vi "SR1.vi"(1 "Spoken text box":refnum<vi>, 2 "new reference":refnum<k24>) -> (0 "事件回调":refnum<k27>)   [LabVIEW 2009]
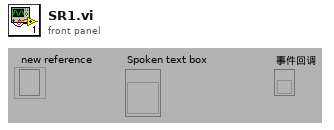
[diagram p1: front panel]
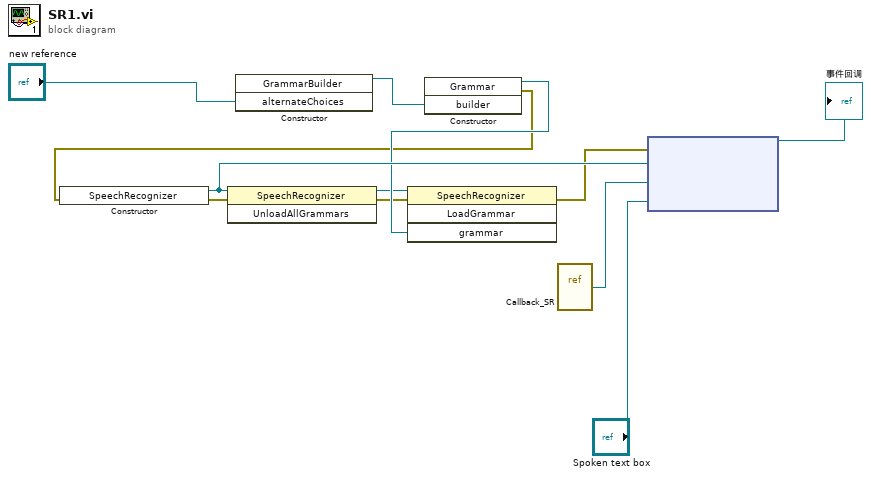
[diagram p0: block diagram]
diagram:
  n1 = constructor class="GrammarBuilder"("alternateChoices"="new reference") -> (reference out=w2:refnum<k24>)  [unwired: 3 in, 3 out]
  n2 = constructor class="Grammar"("builder"=w2) -> (reference out=w7:refnum<k24>, error out=w4:errorcluster)  [unwired: 3 in, 2 out]
  n3 = constructor class="SpeechRecognizer"(error in=w4) -> (reference out=w12:refnum<k24>, error out=w3:errorcluster)  [unwired: 2 in, 1 out]
  n4 = invoke class="SpeechRecognizer" method="UnloadAllGrammars"(reference=w12, error in=w3) -> (reference out=w5:refnum<k24>, error out=w6:errorcluster)  [unwired: 1 in, 1 out]
  n5 = invoke class="SpeechRecognizer" method="LoadGrammar"(reference=w5, error in=w6, "grammar"=w7) -> (error out=w10:errorcluster)  [unwired: 1 in, 3 out]
  n6 = vi-ref "Callback_SR.vi"() -> ("vi reference"=w11:refnum<vi>)
  n7 = node(w10, w12, w11, "Spoken text box") -> (→"事件回调":refnum<k27>)  [unwired: 1 in, 1 out]
